vi "CloseCom6.vi"   [LabVIEW 2023]
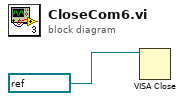
[diagram p0: block diagram]
diagram:
  n1 = VISA Close(VISA resource name=refnum<visa-resource-name> "COM6") -> ()  [unwired: 1 in, 1 out]
